vi "get_material_parameters_cluster.vi"(8 "error in (no error)":errorcluster, 10 "Material number":u8, 11 "VISA resource name":refnum<visa-resource-name>) -> (0 "error out":errorcluster, 2 "Material parameters":T1, 3 "VISA resource name out":refnum<visa-resource-name>)   [LabVIEW 2018]
doc: "Set the density of a material."
uses:
  Low Level/material_parameter_enum.ctl
  Low Level/material_parameters_strings.ctl
  Low Level/material_parameters.ctl
panel:
  in  "Material parameters (strings)":T2
  in  "Material parameter":T3
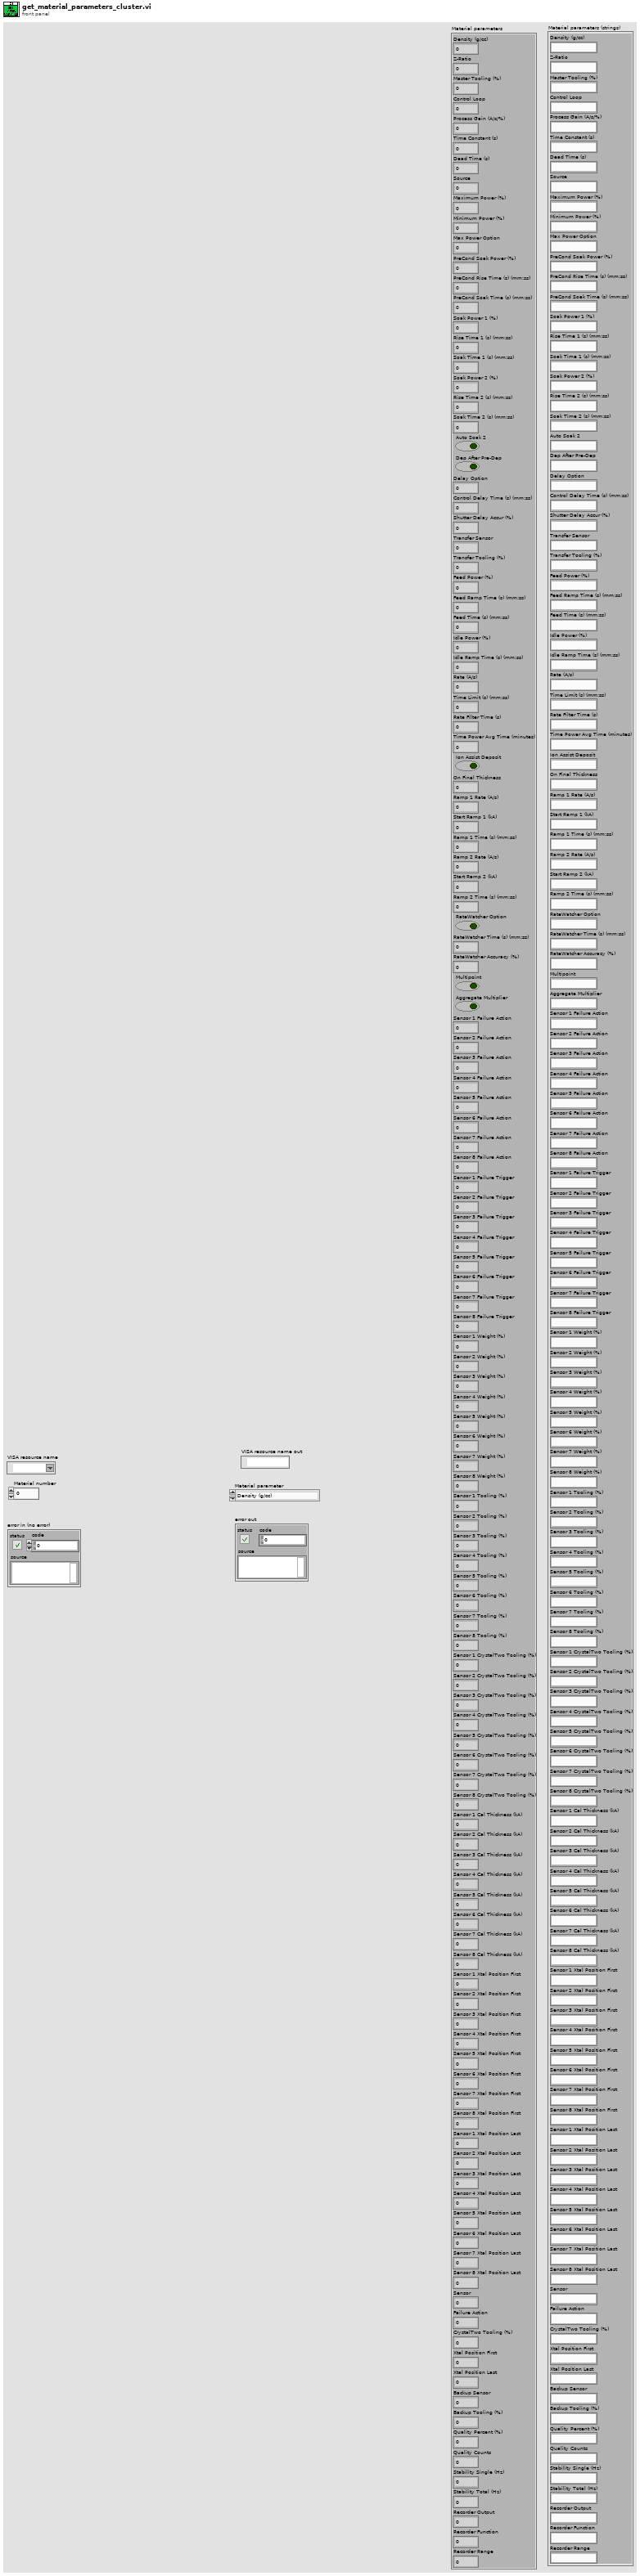
[diagram p1: front panel]
types:
  T1 = typedef "material_parameters.ctl" = cluster{"Density (g/cc)":dbl, "Z-Ratio":dbl, "Master Tooling (%)":dbl, "Control Loop":u8, "Process Gain (A/s/%)":dbl, "Time Constant (s)":dbl, "Dead Time (s)":dbl, "Source":u8, "Maximum Power (%)":dbl, "Minimum Power (%)":dbl, "Max Power Option":u8, "PreCond Soak Power (%)":dbl, "PreCond Rise Time (s) (mm:ss)":u16, "PreCond Soak Time (s) (mm:ss)":u16, "Soak Power 1 (%)":dbl, "Rise Time 1 (s) (mm:ss)":u16, "Soak Time 1 (s) (mm:ss)":u16, "Soak Power 2 (%)":dbl, "Rise Time 2 (s) (mm:ss)":u16, "Soak Time 2 (s) (mm:ss)":u16, "Auto Soak 2":bool, "Dep After Pre-Dep":bool, "Delay Option":u8, "Control Delay Time (s) (mm:ss)":u16, "Shutter Delay Accur (%)":u8, "Transfer Sensor":u8, "Transfer Tooling (%)":dbl, "Feed Power (%)":dbl, "Feed Ramp Time (s) (mm:ss)":u16, "Feed Time (s) (mm:ss)":u16, "Idle Power (%)":dbl, "Idle Ramp Time (s) (mm:ss)":u16, "Rate (A/s)":dbl, "Time Limit (s) (mm:ss)":u16, "Rate Filter Time (s)":u8, "Time Power Avg Time (minutes)":u8, "Ion Assist Deposit":bool, "On Final Thickness":u8, "Ramp 1 Rate (A/s)":dbl, "Start Ramp 1 (kA)":dbl, "Ramp 1 Time (s) (mm:ss)":u16, "Ramp 2 Rate (A/s)":dbl, "Start Ramp 2 (kA)":dbl, "Ramp 2 Time (s) (mm:ss)":u16, "RateWatcher Option":bool, "RateWatcher Time (s) (mm:ss)":u16, "RateWatcher Accuracy (%)":u8, "Multipoint":bool, "Aggregate Multiplier":bool, "Sensor 1 Failure Action":u8, "Sensor 2 Failure Action":u8, "Sensor 3 Failure Action":u8, "Sensor 4 Failure Action":u8, "Sensor 5 Failure Action":u8, "Sensor 6 Failure Action":u8, "Sensor 7 Failure Action":u8, "Sensor 8 Failure Action":u8, "Sensor 1 Failure Trigger":u8, "Sensor 2 Failure Trigger":u8, "Sensor 3 Failure Trigger":u8, "Sensor 4 Failure Trigger":u8, "Sensor 5 Failure Trigger":u8, "Sensor 6 Failure Trigger":u8, "Sensor 7 Failure Trigger":u8, "Sensor 8 Failure Trigger":u8, "Sensor 1 Weight (%)":dbl, "Sensor 2 Weight (%)":dbl, "Sensor 3 Weight (%)":dbl, "Sensor 4 Weight (%)":dbl, "Sensor 5 Weight (%)":dbl, "Sensor 6 Weight (%)":dbl, "Sensor 7 Weight (%)":dbl, "Sensor 8 Weight (%)":dbl, "Sensor 1 Tooling (%)":dbl, "Sensor 2 Tooling (%)":dbl, "Sensor 3 Tooling (%)":dbl, "Sensor 4 Tooling (%)":dbl, "Sensor 5 Tooling (%)":dbl, "Sensor 6 Tooling (%)":dbl, "Sensor 7 Tooling (%)":dbl, "Sensor 8 Tooling (%)":dbl, "Sensor 1 CrystalTwo Tooling (%)":dbl, "Sensor 2 CrystalTwo Tooling (%)":dbl, "Sensor 3 CrystalTwo Tooling (%)":dbl, "Sensor 4 CrystalTwo Tooling (%)":dbl, "Sensor 5 CrystalTwo Tooling (%)":dbl, "Sensor 6 CrystalTwo Tooling (%)":dbl, "Sensor 7 CrystalTwo Tooling (%)":dbl, "Sensor 8 CrystalTwo Tooling (%)":dbl, "Sensor 1 Cal Thickness (kA)":dbl, "Sensor 2 Cal Thickness (kA)":dbl, "Sensor 3 Cal Thickness (kA)":dbl, "Sensor 4 Cal Thickness (kA)":dbl, "Sensor 5 Cal Thickness (kA)":dbl, "Sensor 6 Cal Thickness (kA)":dbl, "Sensor 7 Cal Thickness (kA)":dbl, "Sensor 8 Cal Thickness (kA)":dbl, "Sensor 1 Xtal Position First":u8, "Sensor 2 Xtal Position First":u8, "Sensor 3 Xtal Position First":u8, "Sensor 4 Xtal Position First":u8, "Sensor 5 Xtal Position First":u8, "Sensor 6 Xtal Position First":u8, "Sensor 7 Xtal Position First":u8, "Sensor 8 Xtal Position First":u8, "Sensor 1 Xtal Position Last":u8, "Sensor 2 Xtal Position Last":u8, "Sensor 3 Xtal Position Last":u8, "Sensor 4 Xtal Position Last":u8, "Sensor 5 Xtal Position Last":u8, "Sensor 6 Xtal Position Last":u8, "Sensor 7 Xtal Position Last":u8, "Sensor 8 Xtal Position Last":u8, "Sensor":u8, "Failure Action":u8, "CrystalTwo Tooling (%)":dbl, "Xtal Position First":u8, "Xtal Position Last":u8, "Backup Sensor":u8, "Backup Tooling (%)":dbl, "Quality Percent (%)":u8, "Quality Counts":u8, "Stability Single (Hz)":u8, "Stability Total (Hz)":u8, "Recorder Output":u8, "Recorder Function":u8, "Recorder Range":u8}
  T2 = typedef "material_parameters_strings.ctl" = cluster{"Density (g/cc)":string, "Z-Ratio":string, "Master Tooling (%)":string, "Control Loop":string, "Process Gain (A/s/%)":string, "Time Constant (s)":string, "Dead Time (s)":string, "Source":string, "Maximum Power (%)":string, "Minimum Power (%)":string, "Max Power Option":string, "PreCond Soak Power (%)":string, "PreCond Rise Time (s) (mm:ss)":string, "PreCond Soak Time (s) (mm:ss)":string, "Soak Power 1 (%)":string, "Rise Time 1 (s) (mm:ss)":string, "Soak Time 1 (s) (mm:ss)":string, "Soak Power 2 (%)":string, "Rise Time 2 (s) (mm:ss)":string, "Soak Time 2 (s) (mm:ss)":string, "Auto Soak 2":string, "Dep After Pre-Dep":string, "Delay Option":string, "Control Delay Time (s) (mm:ss)":string, "Shutter Delay Accur (%)":string, "Transfer Sensor":string, "Transfer Tooling (%)":string, "Feed Power (%)":string, "Feed Ramp Time (s) (mm:ss)":string, "Feed Time (s) (mm:ss)":string, "Idle Power (%)":string, "Idle Ramp Time (s) (mm:ss)":string, "Rate (A/s)":string, "Time Limit (s) (mm:ss)":string, "Rate Filter Time (s)":string, "Time Power Avg Time (minutes)":string, "Ion Assist Deposit":string, "On Final Thickness":string, "Ramp 1 Rate (A/s)":string, "Start Ramp 1 (kA)":string, "Ramp 1 Time (s) (mm:ss)":string, "Ramp 2 Rate (A/s)":string, "Start Ramp 2 (kA)":string, "Ramp 2 Time (s) (mm:ss)":string, "RateWatcher Option":string, "RateWatcher Time (s) (mm:ss)":string, "RateWatcher Accuracy (%)":string, "Multipoint":string, "Aggregate Multiplier":string, "Sensor 1 Failure Action":string, "Sensor 2 Failure Action":string, "Sensor 3 Failure Action":string, "Sensor 4 Failure Action":string, "Sensor 5 Failure Action":string, "Sensor 6 Failure Action":string, "Sensor 7 Failure Action":string, "Sensor 8 Failure Action":string, "Sensor 1 Failure Trigger":string, "Sensor 2 Failure Trigger":string, "Sensor 3 Failure Trigger":string, "Sensor 4 Failure Trigger":string, "Sensor 5 Failure Trigger":string, "Sensor 6 Failure Trigger":string, "Sensor 7 Failure Trigger":string, "Sensor 8 Failure Trigger":string, "Sensor 1 Weight (%)":string, "Sensor 2 Weight (%)":string, "Sensor 3 Weight (%)":string, "Sensor 4 Weight (%)":string, "Sensor 5 Weight (%)":string, "Sensor 6 Weight (%)":string, "Sensor 7 Weight (%)":string, "Sensor 8 Weight (%)":string, "Sensor 1 Tooling (%)":string, "Sensor 2 Tooling (%)":string, "Sensor 3 Tooling (%)":string, "Sensor 4 Tooling (%)":string, "Sensor 5 Tooling (%)":string, "Sensor 6 Tooling (%)":string, "Sensor 7 Tooling (%)":string, "Sensor 8 Tooling (%)":string, "Sensor 1 CrystalTwo Tooling (%)":string, "Sensor 2 CrystalTwo Tooling (%)":string, "Sensor 3 CrystalTwo Tooling (%)":string, "Sensor 4 CrystalTwo Tooling (%)":string, "Sensor 5 CrystalTwo Tooling (%)":string, "Sensor 6 CrystalTwo Tooling (%)":string, "Sensor 7 CrystalTwo Tooling (%)":string, "Sensor 8 CrystalTwo Tooling (%)":string, "Sensor 1 Cal Thickness (kA)":string, "Sensor 2 Cal Thickness (kA)":string, "Sensor 3 Cal Thickness (kA)":string, "Sensor 4 Cal Thickness (kA)":string, "Sensor 5 Cal Thickness (kA)":string, "Sensor 6 Cal Thickness (kA)":string, "Sensor 7 Cal Thickness (kA)":string, "Sensor 8 Cal Thickness (kA)":string, "Sensor 1 Xtal Position First":string, "Sensor 2 Xtal Position First":string, "Sensor 3 Xtal Position First":string, "Sensor 4 Xtal Position First":string, "Sensor 5 Xtal Position First":string, "Sensor 6 Xtal Position First":string, "Sensor 7 Xtal Position First":string, "Sensor 8 Xtal Position First":string, "Sensor 1 Xtal Position Last":string, "Sensor 2 Xtal Position Last":string, "Sensor 3 Xtal Position Last":string, "Sensor 4 Xtal Position Last":string, "Sensor 5 Xtal Position Last":string, "Sensor 6 Xtal Position Last":string, "Sensor 7 Xtal Position Last":string, "Sensor 8 Xtal Position Last":string, "Sensor":string, "Failure Action":string, "CrystalTwo Tooling (%)":string, "Xtal Position First":string, "Xtal Position Last":string, "Backup Sensor":string, "Backup Tooling (%)":string, "Quality Percent (%)":string, "Quality Counts":string, "Stability Single (Hz)":string, "Stability Total (Hz)":string, "Recorder Output":string, "Recorder Function":string, "Recorder Range":string}
  T3 = typedef "material_parameter_enum.ctl" = enum16{"Density (g/cc)", "Z-Ratio", "Master Tooling (%)", "Control Loop", "Process Gain (A/s/%)", "Time Constant (s)", "Dead Time (s)", "Source", "Maximum Power (%)", "Minimum Power (%)", "Max Power Option", "PreCond Soak Power (%)", "PreCond Rise Time (s) (mm:ss)", "PreCond Soak Time (s) (mm:ss)", "Soak Power 1 (%)", "Rise Time 1 (s) (mm:ss)", "Soak Time 1 (s) (mm:ss)", "Soak Power 2 (%)", "Rise Time 2 (s) (mm:ss)", "Soak Time 2 (s) (mm:ss)", "Auto Soak 2", "Dep After Pre-Dep", "Delay Option", "Control Delay Time (s) (mm:ss)", "Shutter Delay Accur (%)", "Transfer Sensor", "Transfer Tooling (%)", "Feed Power (%)", "Feed Ramp Time (s) (mm:ss)", "Feed Time (s) (mm:ss)", "Idle Power (%)", "Idle Ramp Time (s) (mm:ss)", "Rate (A/s)", "Time Limit (s) (mm:ss)", "Rate Filter Time (s)", "Time Power Avg Time (minutes)", "Ion Assist Deposit", "On Final Thickness", "Ramp 1 Rate (A/s)", "Start Ramp 1 (kA)", "Ramp 1 Time (s) (mm:ss)", "Ramp 2 Rate (A/s)", "Start Ramp 2 (kA)", "Ramp 2 Time (s) (mm:ss)", "RateWatcher Option", "RateWatcher Time (s) (mm:ss)", "RateWatcher Accuracy (%)", "Multipoint", "Aggregate Multiplier", "Sensor 1 Failure Action", "Sensor 2 Failure Action", "Sensor 3 Failure Action", "Sensor 4 Failure Action", "Sensor 5 Failure Action", "Sensor 6 Failure Action", "Sensor 7 Failure Action", "Sensor 8 Failure Action", "Sensor 1 Failure Trigger", "Sensor 2 Failure Trigger", "Sensor 3 Failure Trigger", "Sensor 4 Failure Trigger", "Sensor 5 Failure Trigger", "Sensor 6 Failure Trigger", "Sensor 7 Failure Trigger", "Sensor 8 Failure Trigger", "Sensor 1 Weight (%)", "Sensor 2 Weight (%)", "Sensor 3 Weight (%)", "Sensor 4 Weight (%)", "Sensor 5 Weight (%)", "Sensor 6 Weight (%)", "Sensor 7 Weight (%)", "Sensor 8 Weight (%)", "Sensor 1 Tooling (%)", "Sensor 2 Tooling (%)", "Sensor 3 Tooling (%)", "Sensor 4 Tooling (%)", "Sensor 5 Tooling (%)", "Sensor 6 Tooling (%)", "Sensor 7 Tooling (%)", "Sensor 8 Tooling (%)", "Sensor 1 CrystalTwo Tooling (%)", "Sensor 2 CrystalTwo Tooling (%)", "Sensor 3 CrystalTwo Tooling (%)", "Sensor 4 CrystalTwo Tooling (%)", "Sensor 5 CrystalTwo Tooling (%)", "Sensor 6 CrystalTwo Tooling (%)", "Sensor 7 CrystalTwo Tooling (%)", "Sensor 8 CrystalTwo Tooling (%)", "Sensor 1 Cal Thickness (kA)", "Sensor 2 Cal Thickness (kA)", "Sensor 3 Cal Thickness (kA)", "Sensor 4 Cal Thickness (kA)", "Sensor 5 Cal Thickness (kA)", "Sensor 6 Cal Thickness (kA)", "Sensor 7 Cal Thickness (kA)", "Sensor 8 Cal Thickness (kA)", "Sensor 1 Xtal Position First", "Sensor 2 Xtal Position First", "Sensor 3 Xtal Position First", "Sensor 4 Xtal Position First", "Sensor 5 Xtal Position First", "Sensor 6 Xtal Position First", "Sensor 7 Xtal Position First", "Sensor 8 Xtal Position First", "Sensor 1 Xtal Position Last", "Sensor 2 Xtal Position Last", "Sensor 3 Xtal Position Last", "Sensor 4 Xtal Position Last", "Sensor 5 Xtal Position Last", "Sensor 6 Xtal Position Last", "Sensor 7 Xtal Position Last", "Sensor 8 Xtal Position Last", "Sensor", "Failure Action", "CrystalTwo Tooling (%)", "Xtal Position First", "Xtal Position Last", "Backup Sensor", "Backup Tooling (%)", "Quality Percent (%)", "Quality Counts", "Stability Single (Hz)", "Stability Total (Hz)", "Recorder Output", "Recorder Function", "Recorder Range"}
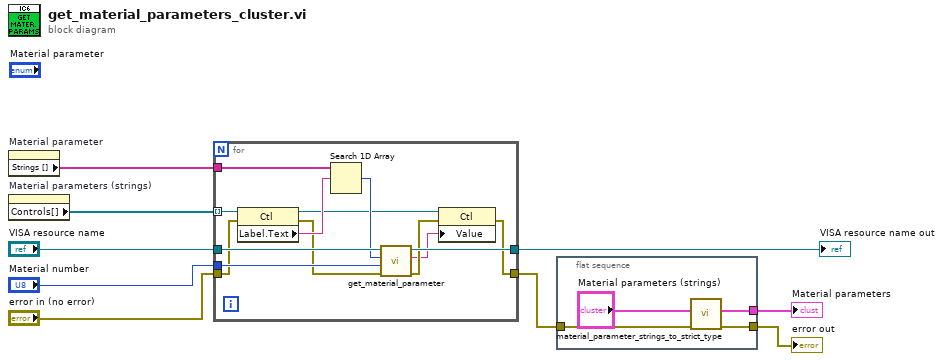
[diagram p0: block diagram]
diagram:
  n1 = property on="Material parameter" class="Enum (strict)"() -> ("Strings []"=w5:string[])  [unwired: 2 in, 2 out]
  n2 = property on="Material parameters (strings)" class="Clust (strict)"() -> ("Controls[]"=w4:refnum<vi>[])  [unwired: 2 in, 2 out]
  n3 = for {
    tunnel: "VISA resource name" -> [w22]
    tunnel: [w21] -> w8
    tunnel: [w10] -> w2
    tunnel: "error in (no error)" -> [w15]
    tunnel: "Material number" -> [w20]
    tunnel: w5 -> [w19]
    tunnel: w4 -> [w18] mode=indexing
    n4 = property class="Ctl"(reference=w18, error in=w15) -> (reference out=w13:refnum<vi>, error out=w14:errorcluster, "Label.Text"=w17:string)
    n5 = Search 1D Array(1D array=w19, element=w17) -> (index of element=w16:i32)  [unwired: 1 in]
    n6 = call "get_material_parameter.vi"("error in (no error)"=w14, "Material number"=w20, "Material parameter"=w16, "VISA resource name"=w22) -> ("error out"=w12:errorcluster, "Material parameter value"=w11:string, "VISA resource name out"=w21:refnum<visa-resource-name>)  [unwired: 5 in]
    n7 = property class="Ctl"(reference=w13, error in=w12, "Value"=w11) -> (error out=w10:errorcluster)  [unwired: 1 out]
  }
  "VISA resource name out" <- w8
  n8 = flat-sequence {
    tunnel: [w24] -> w3
    tunnel: w2 -> [w25]
    tunnel: [w23] -> w1
    frame #0 {
      n9 = call "material_parameter_strings_to_strict_type.vi"("error in (no error)"=w25, "Material parameters (strings)"="Material parameters (strings)") -> ("error out"=w24:errorcluster, "Material parameters"=w23:T1)  [unwired: 8 in]
    }
  }
  "error out" <- w3
  "Material parameters" <- w1
